vi "readFromSerialPort.vi"(2 "Cmmd":string="*idn?", 3 "input COM Port":refnum<visa-resource-name>="COM10") -> (0 "data written to port?":bool=TRUE, 1 "read buffer":string="\n")   [LabVIEW 2015]
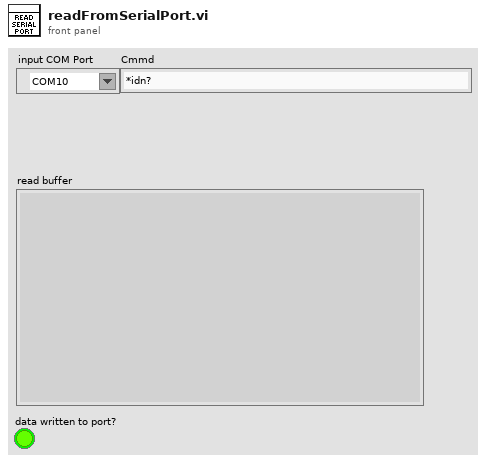
[diagram p1: front panel]
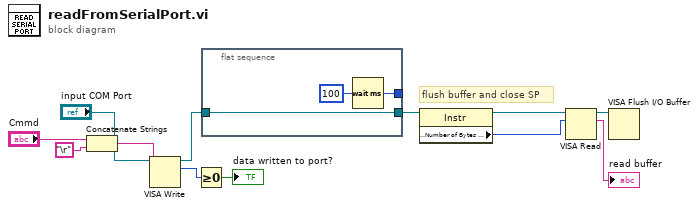
[diagram p0: block diagram]
diagram:
  # "flush buffer and close SP"
  n1 = Concatenate Strings("Cmmd", "\r") -> (w12:string)
  n2 = VISA Write(VISA resource name="input COM Port", write buffer=w12) -> (VISA resource name out=w10:refnum<visa-resource-name>, return count=w8:u32)  [unwired: 1 in, 1 out]
  n3 = Greater Or Equal To 0?(x=w8) -> (x >= 0?=→"data written to port?":bool)
  n4 = flat-sequence {
    tunnel: w10 -> [w15]
    tunnel: [w15] -> w3
    tunnel: [w14] -> _
    frame #0 {
      n5 = Wait (ms)(milliseconds to wait=u32 100) -> (millisecond timer value=w14:u32)
    }
  }
  n6 = property class="Instr"(reference=w3) -> (reference out=w2:refnum<visa-resource-name>, "Serial Settings:Number of Bytes at Serial Port"=w4:u32)  [unwired: 1 in, 1 out]
  n7 = VISA Read(VISA resource name=w2, byte count=w4) -> (VISA resource name out=w1:refnum<visa-resource-name>, read buffer=→"read buffer":string)  [unwired: 1 in, 2 out]
  n8 = VISA Flush I/O Buffer(VISA resource name=w1) -> ()  [unwired: 2 in, 2 out]
